vi "4024_Module_INIT_configure.vi"() -> ()   [LabVIEW 2020]
panel:
  in  "Port Name":string="COM10"
  in  "Slew Rate":u8(ring) items=["Instant", "0.0625 V/sec", "0.125 V/sec", "0.250 V/sec", "0.500 V/sec", "1.000 V/sec", "2.000 V/sec", "4.000 V/sec", "8.000 V/sec", "16.000 V/sec", "32.000 V/sec", "64.000 V/sec"]
  in  "Baud Rate (9600)":u16(ring)=3 items=["1200 bps", "2400 bps", "4800 bps", "9600 bps", "19.2 kbps", "38.4 kbps"]
  in  "Data Format":u8(ring) items=["Engineering Units", "% of FSR", "Hex", "Ohms (4013)"]
  out "Reply":string
  in  "Checksum":bool=TRUE
  out "ConfigStringSent":string
  in  "New Address":u8=196
  in  "Current Address":u8
  # "Run This vi when the the ADAM 4024 is in the INIT mode to set the module address"
  # "Happy reply starts \"!\"\nUnhappy reply starts \"?\""
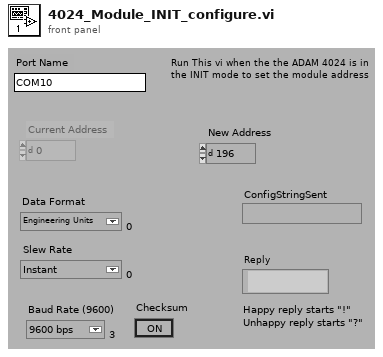
[diagram p1: front panel]
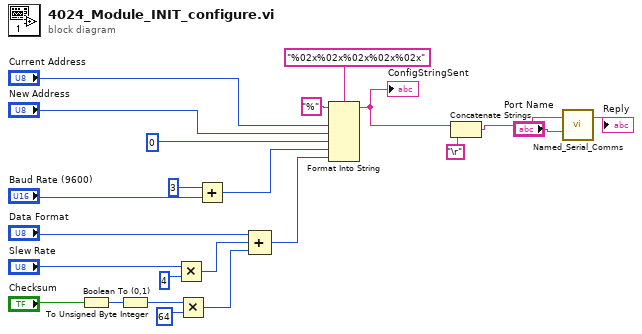
[diagram p0: block diagram]
diagram:
  n1 = Boolean To (0,1)(Boolean="Checksum") -> (0, 1=w8:i16)
  n2 = To Unsigned Byte Integer(number=w8) -> (unsigned 8bit integer=w5:u8)
  n3 = Multiply(x="Slew Rate", y=u8 4) -> (x*y=w10:u8)
  n4 = Multiply(x=w5, y=u8 64) -> (x*y=w6:u8)
  n5 = Add(x=u16 3, y="Baud Rate (9600)") -> (x+y=w16:u16)
  n6 = Compound Arithmetic op=ADD("Data Format", w10, w6) -> (w4:u8)
  n7 = Format Into String(format string="%02x%02x%02x%02x%02x", initial string="%", "Current Address", "New Address", u8 0 ("New Address"), w16, w4) -> (resulting string=w19:string)  [unwired: 1 in, 1 out]
  "ConfigStringSent" <- w19
  n8 = Concatenate Strings(w19, "\r") -> (w14:string)
  n9 = call "Named_Serial_Comms.vi"("Write"=w14, "Port Name"="Port Name") -> ("Read"=→"Reply":string)  [unwired: 9 in, 4 out]
